vi "EMI_projectv2.vi"() -> ()   [LabVIEW 2020]
uses:
  <vilib>/Instr/_visa.llb/VISA Flush IO Buffer Mask.ctl
  <vilib>/Instr/_visa.llb/VISA Configure Serial Port (Instr).vi
panel:
  in  "Slide":dbl(slide) scale=0.0..10.0
  out "Fader02":dbl
  out "Fader01":dbl
  in  "Calibrate":bool
  in  "stop":bool
  in  "VISA resource name":refnum<visa-resource-name>
  in  "?":bool
  in  "Gain02":bool
  in  "?":bool
  in  "Gain01":bool
  in  "?":bool
  in  "Fader02":bool
  in  "?":bool
  in  "Fader01":bool
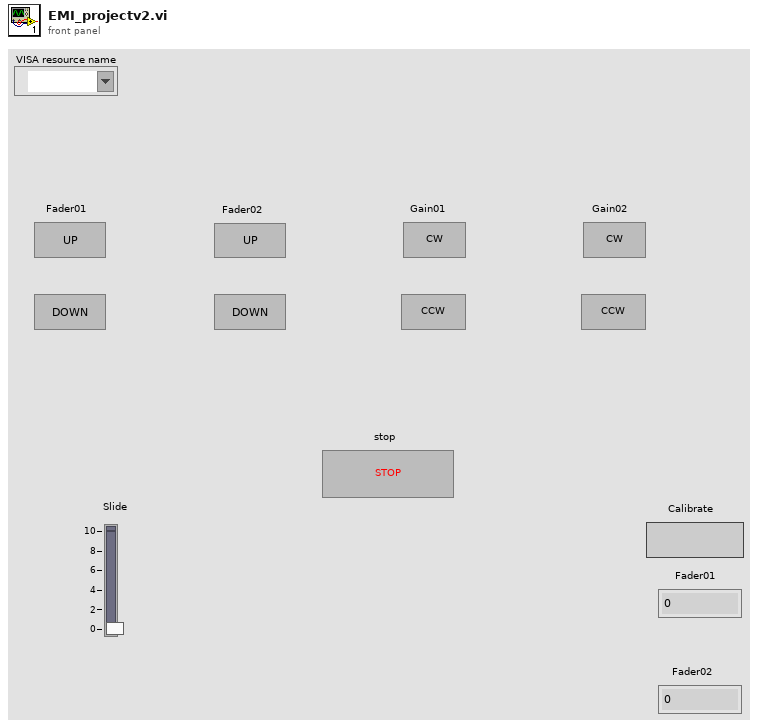
[diagram p1: front panel]
types:
  T1 = typedef "VISA Flush IO Buffer Mask.ctl" = u16
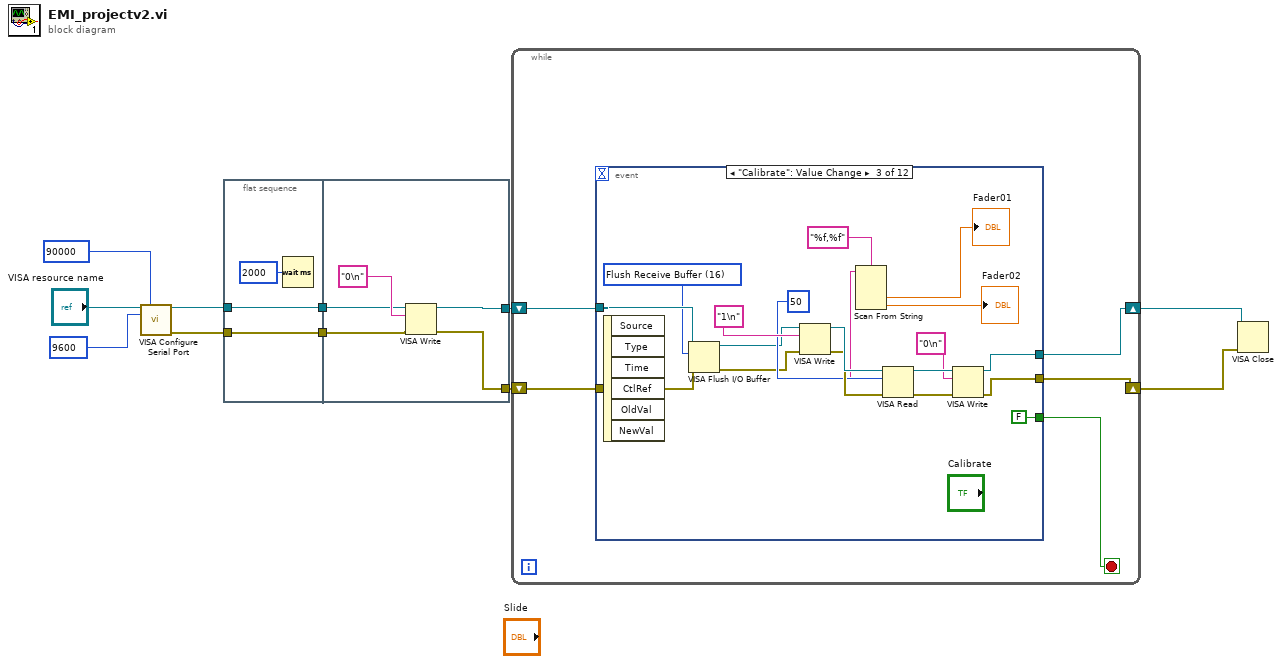
[diagram p0: block diagram]
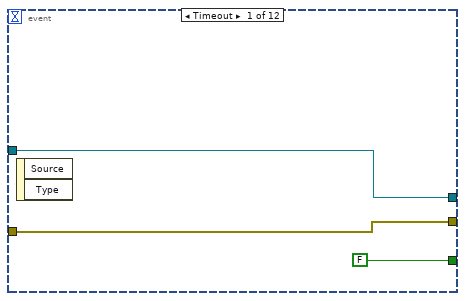
[diagram p2: hidden frame]
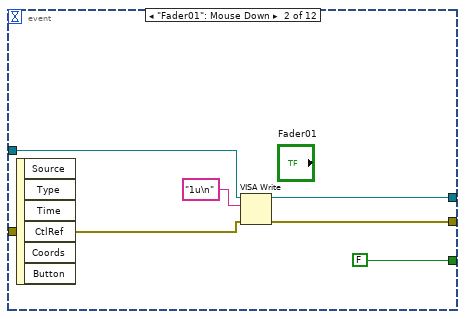
[diagram p3: hidden frame]
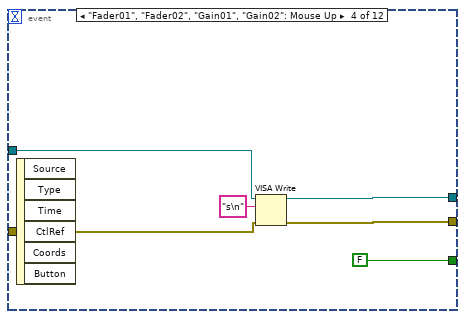
[diagram p4: hidden frame]
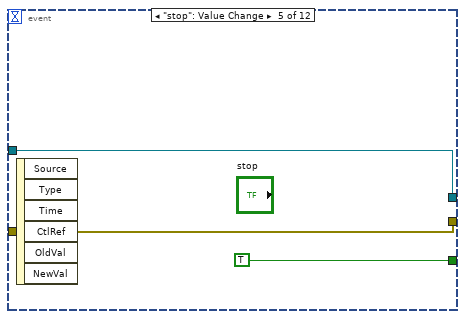
[diagram p5: hidden frame]
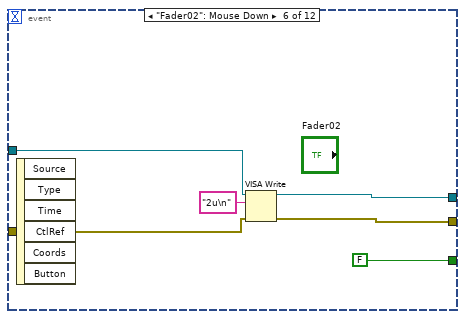
[diagram p6: hidden frame]
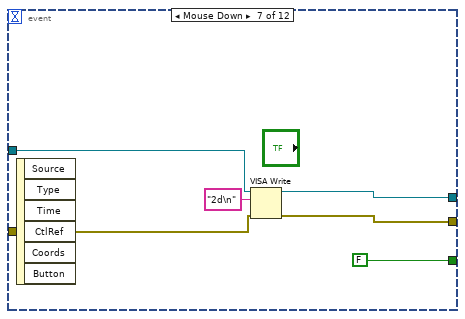
[diagram p7: hidden frame]
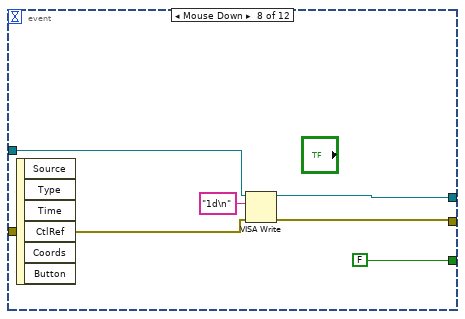
[diagram p8: hidden frame]
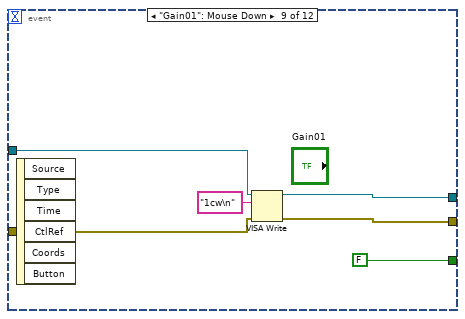
[diagram p9: hidden frame]
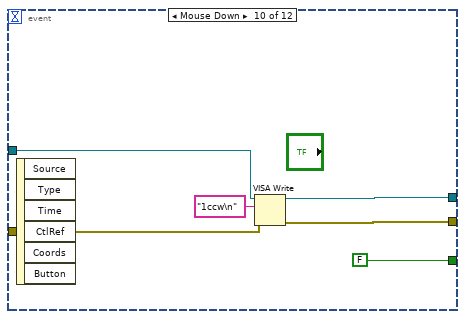
[diagram p10: hidden frame]
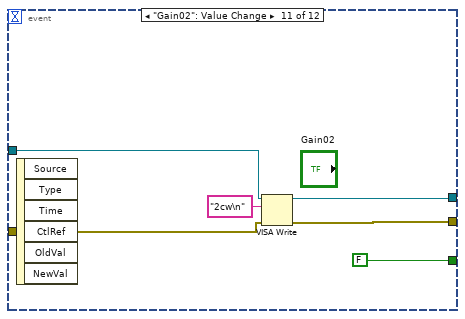
[diagram p11: hidden frame]
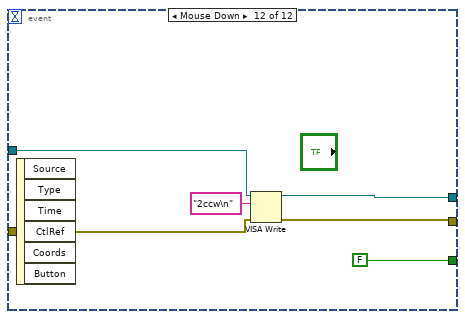
[diagram p12: hidden frame]
diagram:
  n1 = call-poly "VISA Configure Serial Port"("VISA resource name"="VISA resource name", "timeout (10sec)"=u32 90000, "baud rate (9600)"=u32 9600) -> ("VISA resource name out"=w5:refnum<visa-resource-name>, "error out"=w4:errorcluster)  [unwired: 11 in]
  n2 = flat-sequence {
    tunnel: w4 -> [w13]
    tunnel: w5 -> [w14]
    tunnel: [w14] -> w3
    tunnel: [w13] -> w2
    tunnel: [w18] -> w9
    tunnel: [w17] -> w8
    tunnel: w3 -> [w16]
    tunnel: w2 -> [w15]
    frame #0 {
      n3 = Wait (ms)(milliseconds to wait=u32 2000) -> ()  [unwired: 1 out]
    }
    frame #1 {
      n4 = VISA Write(VISA resource name=w16, write buffer="0\n", error in (no error)=w15) -> (VISA resource name out=w18:refnum<visa-resource-name>, error out=w17:errorcluster)  [unwired: 1 out]
    }
  }
  n5 = while {
    shift-right: [w22] -> w7
    shift-left: w9 -> [w24]
    shift-right: [w21] -> w6
    shift-left: w8 -> [w23]
    stop <- w20 stop-if-true
    n6 = event shown="[2] \"Calibrate\": Value Change" {
      selector: _ -> [_ _ _ _ _ _ _ _ _ _ _ _]
      dyn-events: _ -> [_ _ _ _ _ _ _ _ _ _ _ _]
      timeout: _ -> [_ _ _ _ _ _ _ _ _ _ _ _]
      tunnel: w24 -> [w27 w33 w43 w56 w60 w65 w71 w79 w83 w88 w95 w101]
      tunnel: w23 -> [w26 w32 w42 w55 w59 w64 w70 w78 w82 w89 w94 w100]
      tunnel: [w27 w30 w35 w58 w60 w67 w73 w76 w85 w91 w97 w103] -> w22
      tunnel: [w26 w29 w36 w57 w59 w66 w72 w77 w84 w90 w96 w102] -> w21
      tunnel: [FALSE FALSE FALSE FALSE TRUE FALSE FALSE FALSE FALSE FALSE FALSE FALSE] -> w20
      event Timeout {
        n7 = event-data() -> ()  [unwired: 1 in, 2 out]
      }
      event "Fader01": Mouse Down {
        n8 = event-data() -> ()  [unwired: 1 in, 6 out]
        n9 = VISA Write(VISA resource name=w33, write buffer="1u\n", error in (no error)=w32) -> (VISA resource name out=w30:refnum<visa-resource-name>, error out=w29:errorcluster)  [unwired: 1 out]
      }
      event "Calibrate": Value Change {
        w39 = T1 16 items=["Flush Receive Buffer"=16, "Write Transmit Buffer to Device"=32, "Flush Receive Buffer (No I/O)"=64, "Flush Transmit Buffer"=128] ("Mask")
        n10 = event-data() -> ()  [unwired: 1 in, 6 out]
        n11 = VISA Flush I/O Buffer(VISA resource name=w43, mask (16)=w39, error in (no error)=w42) -> (VISA resource name out=w41:refnum<visa-resource-name>, error out=w40:errorcluster)
        n12 = VISA Write(VISA resource name=w41, write buffer="1\n", error in (no error)=w40) -> (VISA resource name out=w51:refnum<visa-resource-name>, error out=w50:errorcluster)  [unwired: 1 out]
        n13 = VISA Read(VISA resource name=w51, byte count=u32 50, error in (no error)=w50) -> (VISA resource name out=w38:refnum<visa-resource-name>, read buffer=w48:string, error out=w37:errorcluster)  [unwired: 1 out]
        n14 = Scan From String(format string="%f,%f", input string=w48) -> (output 1=→"Fader01":dbl, output 2=→"Fader02":dbl)  [unwired: 4 in, 3 out]
        n15 = VISA Write(VISA resource name=w38, write buffer="0\n", error in (no error)=w37) -> (VISA resource name out=w35:refnum<visa-resource-name>, error out=w36:errorcluster)  [unwired: 1 out]
      }
      event "Fader01", "Fader02", "Gain01", "Gain02": Mouse Up {
        n16 = event-data() -> ()  [unwired: 1 in, 6 out]
        n17 = VISA Write(VISA resource name=w56, write buffer="s\n", error in (no error)=w55) -> (VISA resource name out=w58:refnum<visa-resource-name>, error out=w57:errorcluster)  [unwired: 1 out]
      }
      event "stop": Value Change {
        n18 = event-data() -> ()  [unwired: 1 in, 6 out]
      }
      event "Fader02": Mouse Down {
        n19 = event-data() -> ()  [unwired: 1 in, 6 out]
        n20 = VISA Write(VISA resource name=w65, write buffer="2u\n", error in (no error)=w64) -> (VISA resource name out=w67:refnum<visa-resource-name>, error out=w66:errorcluster)  [unwired: 1 out]
      }
      event Mouse Down {
        n21 = event-data() -> ()  [unwired: 1 in, 6 out]
        n22 = VISA Write(VISA resource name=w71, write buffer="2d\n", error in (no error)=w70) -> (VISA resource name out=w73:refnum<visa-resource-name>, error out=w72:errorcluster)  [unwired: 1 out]
      }
      event Mouse Down {
        n23 = event-data() -> ()  [unwired: 1 in, 6 out]
        n24 = VISA Write(VISA resource name=w79, write buffer="1d\n", error in (no error)=w78) -> (VISA resource name out=w76:refnum<visa-resource-name>, error out=w77:errorcluster)  [unwired: 1 out]
      }
      event "Gain01": Mouse Down {
        n25 = event-data() -> ()  [unwired: 1 in, 6 out]
        n26 = VISA Write(VISA resource name=w83, write buffer="1cw\n", error in (no error)=w82) -> (VISA resource name out=w85:refnum<visa-resource-name>, error out=w84:errorcluster)  [unwired: 1 out]
      }
      event Mouse Down {
        n27 = event-data() -> ()  [unwired: 1 in, 6 out]
        n28 = VISA Write(VISA resource name=w88, write buffer="1ccw\n", error in (no error)=w89) -> (VISA resource name out=w91:refnum<visa-resource-name>, error out=w90:errorcluster)  [unwired: 1 out]
      }
      event "Gain02": Value Change {
        n29 = event-data() -> ()  [unwired: 1 in, 6 out]
        n30 = VISA Write(VISA resource name=w95, write buffer="2cw\n", error in (no error)=w94) -> (VISA resource name out=w97:refnum<visa-resource-name>, error out=w96:errorcluster)  [unwired: 1 out]
      }
      event Mouse Down {
        n31 = event-data() -> ()  [unwired: 1 in, 6 out]
        n32 = VISA Write(VISA resource name=w101, write buffer="2ccw\n", error in (no error)=w100) -> (VISA resource name out=w103:refnum<visa-resource-name>, error out=w102:errorcluster)  [unwired: 1 out]
      }
    }
  }
  n33 = VISA Close(VISA resource name=w7, error in (no error)=w6) -> ()  [unwired: 1 out]
